vi "IMS Stepper Wait for Move.vi"(5 "error in (no error)":errorcluster, 7 "Motor Number":u32=1 min=1 max=255 step=1, 8 "Instrument Address":refnum<visa-resource-name>) -> (0 "error out":errorcluster, 3 "Instrument Address Out":refnum<visa-resource-name>)   [LabVIEW 2024]
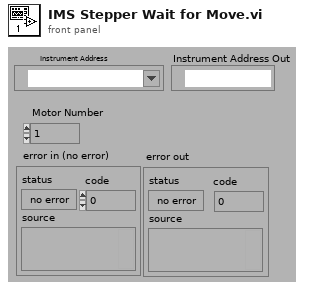
[diagram p1: front panel]
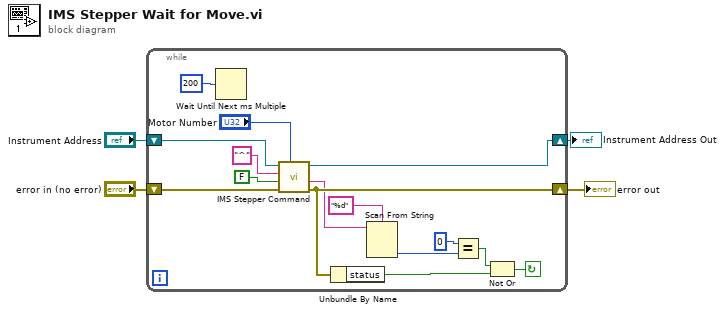
[diagram p0: block diagram]
diagram:
  n1 = while {
    shift-left: "error in (no error)" -> [w16]
    shift-right: [w15] -> w3
    shift-right: [w6] -> w1
    shift-left: "Instrument Address" -> [w5]
    stop <- w14 continue-if-true
    n2 = Wait Until Next ms Multiple(millisecond multiple=u32 200) -> ()  [unwired: 1 out]
    n3 = call "IMS Stepper Command.vi"("Motor Number"="Motor Number", "error in (no error)"=w16, "Mode"=FALSE, "Command"="^", "Instrument Address"=w5) -> ("error out"=w15:errorcluster, "Response"=w9:string, "Instrument Address Out"=w6:refnum<visa-resource-name>)  [unwired: 1 in, 1 out]
    n4 = Unbundle By Name(w15) -> ("status"=w13:bool)
    n5 = Scan From String(format string="%d", input string=w9) -> (output 1=w10:i32)  [unwired: 3 in, 3 out]
    n6 = Equal?(x=0, y=w10) -> (x = y?=w12:bool)
    n7 = Not Or(1:w13, 2:w12) -> (0:w14:bool)
  }
  "error out" <- w3
  "Instrument Address Out" <- w1
